vi "BB Write Target Angle Vertical.vi"(11 "Results":T1 {"Score" format="%#_3g"; "Pixels"."Rectangle"."Numeric 5" format="%#_3g"; "Pixels"."Rectangle"."Numeric 3" format="%#_3g"; "Pixels"."Rectangle"."Numeric 2" format="%#_3g"; "Pixels"."Rectangle"."Numeric" format="%#_3g"; "Normalized"."Rectangle"."Numeric 5" format="%#_2g"; "Normalized"."Rectangle"."Numeric 3" format="%#_2g"; "Normalized"."Rectangle"."Numeric 2" format="%#_2g"; "Normalized"."Rectangle"."Numeric" format="%#_2g"; "Normalized"."Center"."?" format="%#_3g"; "Normalized"."Center"."?" format="%#_3g"; "Distance (ft)" format="%#_3g"}) -> (1 "TargetDistance":dbl, 2 "TargetDetected":bool, 3 "TargetAngle":dbl)   [LabVIEW 2016]
uses:
  Camera Types.ctl
  <vilib>/Rock Robotics/Network Tables/NT Write Boolean.vi
  <vilib>/Rock Robotics/Network Tables/NT Write Number.vi
panel:
  in  "Camera Type":T2=enum."MS HD3000 square"
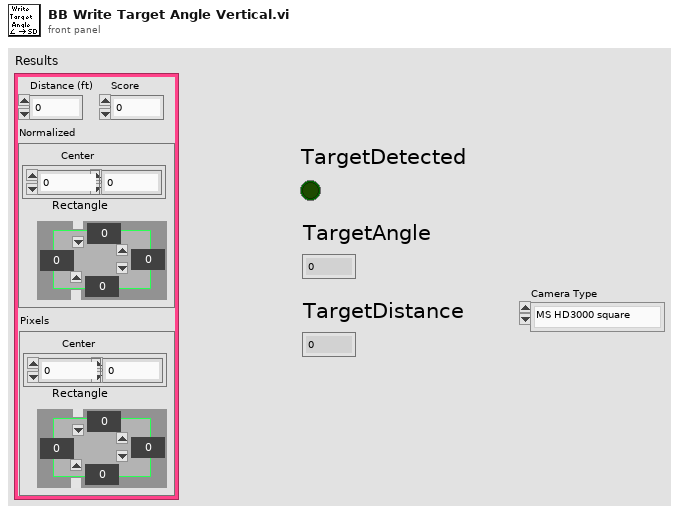
[diagram p1: front panel]
types:
  T1 = cluster{"Distance (ft)":dbl, "Score":dbl, "Normalized":cluster{"Center":cluster{dbl, dbl}, "Rectangle":cluster{"Numeric":dbl, "Numeric 2":dbl, "Numeric 3":dbl, "Numeric 5":dbl}}, "Pixels":cluster{"Center":cluster{dbl, dbl}, "Rectangle":cluster{"Numeric":dbl, "Numeric 2":dbl, "Numeric 3":dbl, "Numeric 5":dbl}}}
  T2 = typedef "Camera Types.ctl" = enum16{"206", "1011", "1013", "MS HD3000 square", "MS HD3000 640x480"}
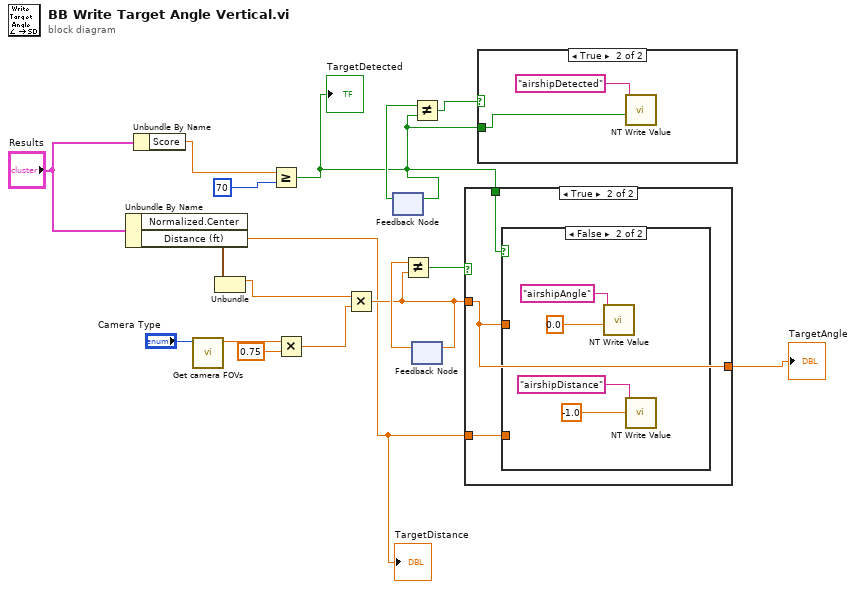
[diagram p0: block diagram]
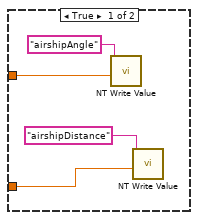
[diagram p4: hidden frame]
diagram:
  n1 = Unbundle By Name("Results") -> ("Normalized.Center"=w17:cluster{dbl, dbl}, "Distance (ft)"=w7:dbl)
  "TargetDistance" <- w7
  n2 = Unbundle By Name("Results") -> ("Score"=w2:dbl)
  n3 = call "Get camera FOVs.vi"("Camera Type"="Camera Type") -> ("FOV"=w15:dbl)  [unwired: 9 in, 1 out]
  n4 = Unbundle(w17) -> (w13:dbl)  [unwired: 1 out]
  n5 = Greater Or Equal?(x=w2, y=70) -> (x >= y?=w1:bool)
  "TargetDetected" <- w1
  n6 = Multiply(x=w15, y=0.75) -> (x*y=w12:dbl)
  n7 = Multiply(x=w13, y=w12) -> (x*y=w10:dbl)
  n8 = feedback #1() -> (w6:bool)  [unwired: 1 in]
  n9 = feedback-in #1(w1) -> ()
  n10 = Not Equal?(x=w6, y=w1) -> (x != y?=w5:bool)
  n11 = feedback-in #2(w10) -> ()
  n12 = feedback #2() -> (w11:dbl)  [unwired: 1 in]
  n13 = Not Equal?(x=w11, y=w10) -> (x != y?=w9:bool)
  n14 = case shown="True" w9 {
    tunnel: w10 -> [w18 w21]
    tunnel: [w18 w21] -> w8
    tunnel: w7 -> [_ w20]
    tunnel: w1 -> [_ w19]
    frame False {
    }
    frame True {
      n15 = case shown="False" w19 {
        tunnel: w21 -> [w24 _]
        tunnel: w20 -> [w23 _]
        frame True {
          n16 = call-poly <vilib>:"NT Write Value.vi"("Numeric"=w24, "Name"="airshipAngle") -> ()  [unwired: 9 in, 1 out]
          n17 = call-poly <vilib>:"NT Write Value.vi"("Numeric"=w23, "Name"="airshipDistance") -> ()  [unwired: 9 in, 1 out]
        }
        frame False {
          n18 = call-poly <vilib>:"NT Write Value.vi"("Numeric"=0.0, "Name"="airshipAngle") -> ()  [unwired: 9 in, 1 out]
          n19 = call-poly <vilib>:"NT Write Value.vi"("Numeric"=-1.0, "Name"="airshipDistance") -> ()  [unwired: 9 in, 1 out]
        }
      }
    }
  }
  "TargetAngle" <- w8
  n20 = case shown="True" w5 {
    tunnel: w1 -> [_ w31]
    frame False {
    }
    frame True {
      n21 = call-poly <vilib>:"NT Write Value.vi"("Boolean"=w31, "Name"="airshipDetected") -> ()  [unwired: 9 in, 1 out]
    }
  }
